vi "DoValve.vi"(6 "#DO":T1[](array[typedef]) items=["DO 0 [KP1] [M12]", "DO 1 [ON KP2] [M21]", "DO 2 [ON KP3] [M24]", "DO 3 [WATER Y18.1 [DO3]]", "DO 4 [WATER Y18.2 [DO4]]", "DO 5 [KP6 Y29.1 33.7]", "DO 6 [KP7 Y29.2 33.8]", "DO 7 [KP8 Y29.3 33.9]", "DO 8 [KP9 Y29.4  33.12]", "DO 9 [KP10 Y29.5 33.1]", "DO 10 [KP11 Y29.6 33.2]", "DO 11 [KP12 Y29.7  33.13]", "DO 12 [KP13 Y29.8  33.11]", "DO 13 [KP14 Y29.9 33.10]", "DO 14 [KP15 Y29.10  33.6]", "DO 15 [KP16 Y29.11  33.5]", "DO 16 [KP17 Y29.12  33.4]", "DO 17 [KP18 Y29.13 33.3]", "DO 18 [AIR KP19]", "DO 19 [STEP DRIVE EN KP20]", "DO 20 [KP21 Y44.1 OPEN]", "DO 21 [ KP22 Y44.1 CLOSE]", "DO 22 [ KP23 Y44.2 OPEN]", "DO 23", "DO 24 [STEP DRIVE 1]", "DO 25 [STEP DRIVE 2]"], 7 "Reset":bool, 8 "error in (no error)":errorcluster, 10 "time after close":i32 caption="Time Target (s)", 11 "reference in":refnum<class "FPGA API.lvclass">) -> (0 "error out":errorcluster, 2 "Done":bool caption="Time has Elapsed", 3 "reference out":refnum<class "FPGA API.lvclass">)   [LabVIEW 2019, in "Stand.lvclass"]
uses:
  Stand.lvclass
  FPGA_API_class/FPGA API.lvclass
  FPGA/TypeDef/DO index.ctl
  e7d2c9dc-ba67-4685-b926-bcce34aa2778.vi
  628819af-fd07-4303-9780-3ddd467101db.vi
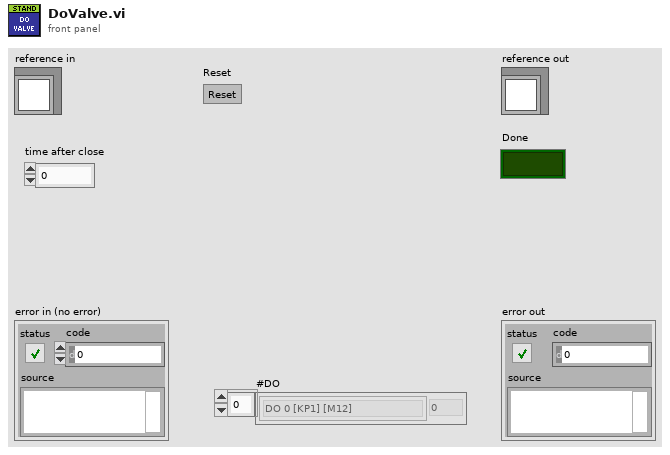
[diagram p1: front panel]
types:
  T1 = typedef "DO index.ctl" = u8
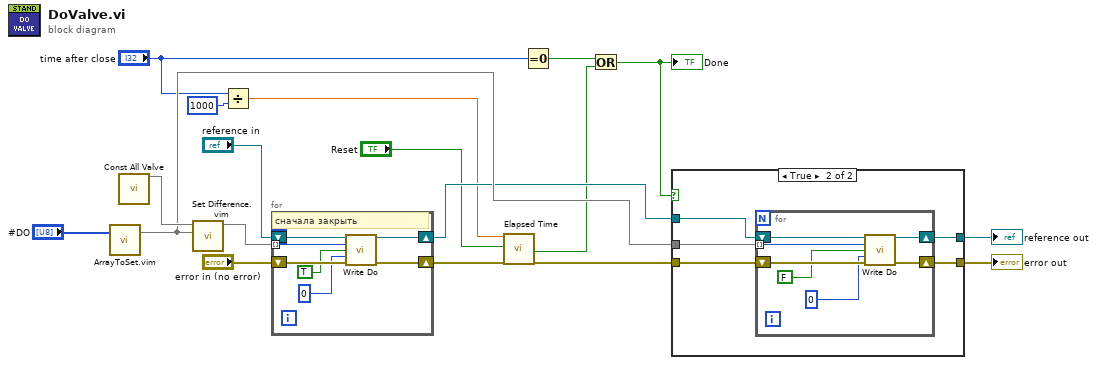
[diagram p0: block diagram]
diagram:
  n1 = call "ArrayToSet.vim"("Array"="#DO") -> ("Set"=w15:set{T1})  [unwired: 2 in]
  n2 = call "Const All Valve.vi"() -> ("Set"=w17:set{T1})  [unwired: 15 in]
  n3 = call "Set Difference.vim"("set 2"=w15, "set 1"=w17) -> ("difference"=w16:set{T1})  [unwired: 9 in]
  n4 = Divide(x="time after close", y=1000 ("x")) -> (x/y=w6:dbl)
  n5 = for {
    shift-right: [w23] -> w8
    shift-left: "error in (no error)" -> [w24]
    tunnel: w16 -> [w22] mode=indexing
    shift-right: [w19] -> w12
    shift-left: "reference in" -> [w25]
    # "сначала закрыть"
    n6 = call-dynamic "Write Do.vi"("FPGA API in"=w25, "#DO"=w22, "value"=TRUE, "Time uSec"=u32 0, "error in (no error)"=w24) -> ("FPGA API out"=w19:refnum<class "FPGA API.lvclass">, "error out"=w23:errorcluster)  [unwired: 9 in]
  }
  n7 = call "Elapsed Time"("Time Target (s)"=w6, "Reset"="Reset", "error in (no error)"=w8) -> ("Time has Elapsed"=w4:bool, "error out"=w7:errorcluster)  [unwired: 9 in, 6 out]
  n8 = Equal To 0?(x="time after close") -> (x = 0?=w1:bool)
  n9 = Or(x=w1, y=w4) -> (x .or. y?=w2:bool)
  "Done" <- w2
  n10 = case shown="True" w2 {
    tunnel: w15 -> [_ w32]
    tunnel: [w26 w31] -> w13
    tunnel: w12 -> [w27 w30]
    tunnel: [w27 w29] -> w11
    tunnel: w7 -> [w26 w28]
    frame False {
    }
    frame True {
      n11 = for {
        shift-right: [w37] -> w31
        shift-left: w28 -> [w38]
        tunnel: w32 -> [w36] mode=indexing
        shift-right: [w34] -> w29
        shift-left: w30 -> [w39]
        n12 = call-dynamic "Write Do.vi"("FPGA API in"=w39, "#DO"=w36, "value"=FALSE, "Time uSec"=u32 0, "error in (no error)"=w38) -> ("FPGA API out"=w34:refnum<class "FPGA API.lvclass">, "error out"=w37:errorcluster)  [unwired: 9 in]
      }
    }
  }
  "error out" <- w13
  "reference out" <- w11
